vi "Get Target Train Field (No Objects).vi"(8 "Train to Field":dbl[unit]=7.0, 9 "Original Field":dbl[unit], 10 "going up?":bool=TRUE, 11 "Cluster In":T4={"Field"=0.0, "Rate"=0.0, "Status"={"Sweeping"=FALSE, "Clamped"=FALSE, "Hold"=FALSE, "At Rest"=FALSE, "Quench"=FALSE, "Persistent Mode"=FALSE, "Switch Heater"=FALSE}, "ILM Shut Down?"=FALSE, "IO Info"={"Address"={"Com Port"=1, "ISOBUS Address"=2, "GPIB Address"=24, "Communication"=enum."ISOBUS"}, "Version"=enum."IPS"}, "IO Info (Level Meter)"={"Address"={"Com Port"=1, "ISOBUS Address"=5, "GPIB Address"=24, "Communication"=enum."ISOBUS"}, "ILM Name"="", "Display Channel"=[]}, "Training?"=FALSE, "Training Field and Speed Cluster"={"Training Field"=[0.0, 4.108, 5.78, 8.001], "Training Speed"=[0.0057, 0.0022833333333333334, 0.0011333333333333334, 0.0011333333333333334]}}) -> (2 "Target Field":dbl[unit], 3 "Cluster Out":T4={"Field"=0.0, "Rate"=0.0, "Status"={"Sweeping"=FALSE, "Clamped"=FALSE, "Hold"=FALSE, "At Rest"=FALSE, "Quench"=FALSE, "Persistent Mode"=FALSE, "Switch Heater"=FALSE}, "ILM Shut Down?"=FALSE, "IO Info"={"Address"={"Com Port"=1, "ISOBUS Address"=2, "GPIB Address"=24, "Communication"=enum."ISOBUS"}, "Version"=enum."IPS"}, "IO Info (Level Meter)"={"Address"={"Com Port"=1, "ISOBUS Address"=5, "GPIB Address"=24, "Communication"=enum."ISOBUS"}, "ILM Name"="", "Display Channel"=[]}, "Training?"=FALSE, "Training Field and Speed Cluster"={"Training Field"=[0.0, 4.108, 5.78, 8.001], "Training Speed"=[0.0057, 0.0022833333333333334, 0.0011333333333333334, 0.0011333333333333334]}})   [LabVIEW 2009]
uses:
  Magnet status.ctl
  Oxford/PSSUBS.LLB/PSIO.ctl
  Oxford/BUSGEN.LLB/OxfordAddress.ctl
  Power Supply.lvclass
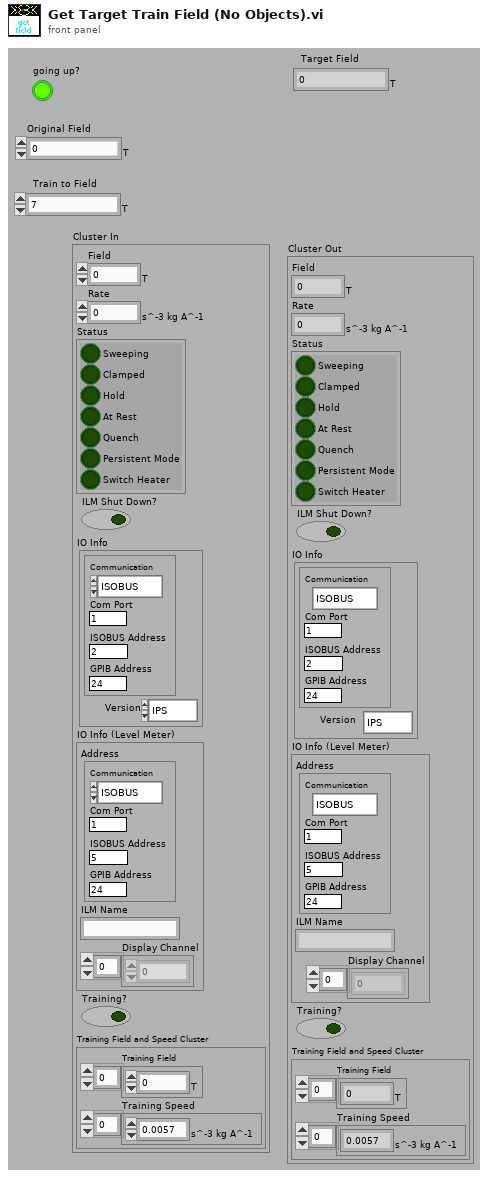
[diagram p1: front panel]
types:
  T1 = typedef "Power Supply.lvclass/Magnet status.ctl" = cluster{"Sweeping":bool, "Clamped":bool, "Hold":bool, "At Rest":bool, "Quench":bool, "Persistent Mode":bool, "Switch Heater":bool}
  T2 = typedef "PSIO.ctl" = cluster{"Address":T3, "Version":enum16{"PS", "IPS"}}
  T3 = typedef "OxfordAddress.ctl" = cluster{"Com Port":i32, "ISOBUS Address":i32, "GPIB Address":i16, "Communication":enum16{"RS232", "ISOBUS", "GPIB", "Gateway"}}
  T4 = cluster{"Field":dbl[unit], "Rate":dbl[unit], "Status":T1, "ILM Shut Down?":bool, "IO Info":T2, "IO Info (Level Meter)":cluster{"Address":T3, "ILM Name":string, "Display Channel":i32[]}, "Training?":bool, "Training Field and Speed Cluster":cluster{"Training Field":dbl[unit][], "Training Speed":dbl[unit][]}}
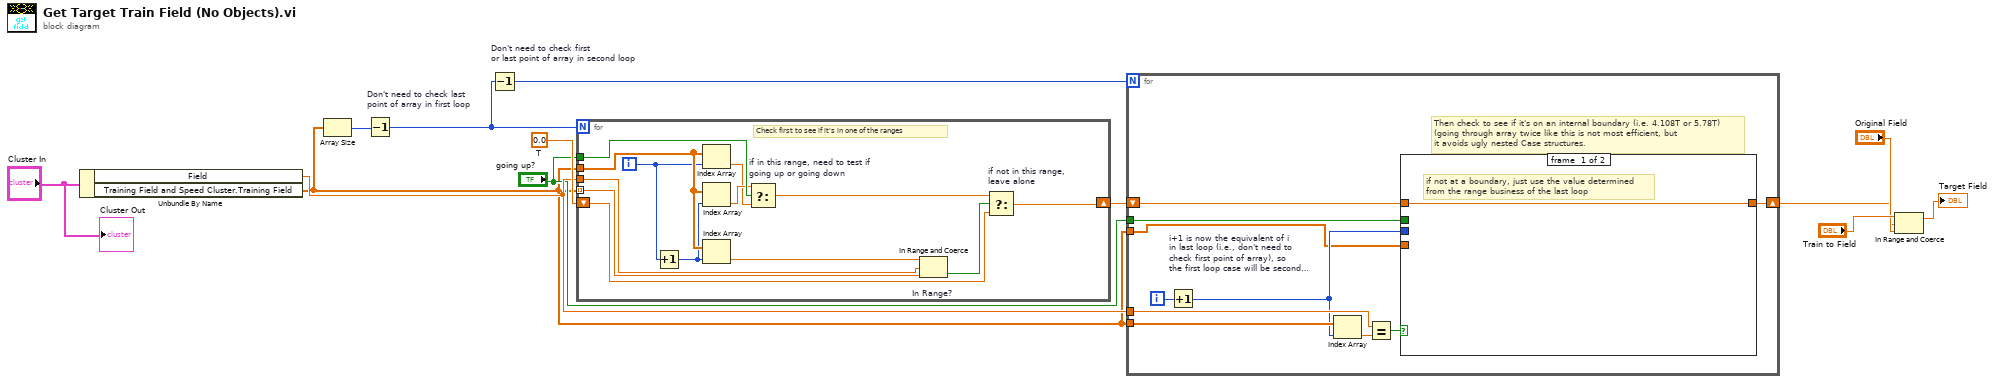
[diagram p0: block diagram]
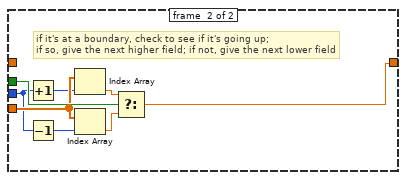
[diagram p2: hidden frame]
diagram:
  w12 = dbl[unit] 0.0  # T
  n1 = Unbundle By Name("Cluster In") -> ("Field"=w9:dbl[unit], "Training Field and Speed Cluster.Training Field"=w6:dbl[unit][])
  n2 = Array Size(array=w6) -> (size(s)=w13:i32)
  n3 = Decrement "Don't need to check last \npoint of array in first loop"(x=w13) -> (x-1=w10:i32)
  n4 = Decrement "Don't need to check first\nor last point of array in second loop"(x=w10) -> (x-1=w8:i32)
  n5 = for {
    N: w10 -> [_]
    tunnel: w9 -> [w25]
    tunnel: w6 -> [w19]
    tunnel: w6 -> [w24] mode=indexing
    shift-right: [w22] -> w11
    shift-left: w12 -> [w21]
    tunnel: "going up?" -> [w20]
    i -> [w17]
    # "Check first to see if it's in one of the ranges"
    n6 = Increment(x=w17) -> (x+1=w18:i32)
    n7 = Index Array(array=w19, index=w17) -> (element=w15:dbl[unit])
    n8 = Index Array(array=w19, index=w18) -> (element=w16:dbl[unit])
    n9 = Index Array(array=w19, index=w18) -> (element=w26:dbl[unit])
    n10 = Select "if in this range, need to test if \ngoing up or going down"(t=w16, s=w20, f=w15) -> (s? t:f=w14:dbl[unit])
    n11 = In Range and Coerce "In Range?"(upper limit=w26, x=w25, lower limit=w24) -> (In Range?=w23:bool)  [unwired: 1 out]
    n12 = Select "if not in this range,\nleave alone"(t=w14, s=w23, f=w21) -> (s? t:f=w22:dbl[unit])
  }
  n13 = for {
    N: w8 -> [_]
    tunnel: w9 -> [w33]
    tunnel: w6 -> [w31]
    shift-right: [w35] -> w2
    shift-left: w11 -> [w34]
    tunnel: "going up?" -> [w28]
    tunnel: w6 -> [w27]
    i -> [w36]
    # "Then check to see if it's on an internal boundary (i.e. 4.108T or 5.78T)\n(going through array twice like this is not most efficient, but\nit avoids ugly nested Case structures."
    n14 = Increment "i+1 is now the equivalent of i\nin last loop (i.e., don't need to \ncheck first point of array), so \nthe first loop case will be second\npoint"(x=w36) -> (x+1=w29:i32)
    n15 = Index Array(array=w31, index=w29) -> (element=w30:dbl[unit])
    n16 = Equal?(x=w33, y=w30) -> (x = y?=w32:bool)
    n17 = case shown="True" w32 {
      tunnel: [w37 w40] -> w35
      tunnel: w34 -> [w37 _]
      tunnel: w29 -> [_ w39]
      tunnel: w28 -> [_ w42]
      tunnel: w27 -> [_ w41]
      frame #0 {
        # "if not at a boundary, just use the value determined \nfrom the range business of the last loop"
      }
      frame #1 {
        # "if it's at a boundary, check to see if it's going up; \nif so, give the next higher field; if not, give the next lower field"
        n18 = Increment(x=w39) -> (x+1=w38:i32)
        n19 = Decrement(x=w39) -> (x-1=w45:i32)
        n20 = Index Array(array=w41, index=w38) -> (element=w44:dbl[unit])
        n21 = Index Array(array=w41, index=w45) -> (element=w43:dbl[unit])
        n22 = Select(t=w44, s=w42, f=w43) -> (s? t:f=w40:dbl[unit])
      }
    }
  }
  n23 = In Range and Coerce(upper limit="Train to Field", x=w2, lower limit="Original Field") -> (coerced(x)=→"Target Field":dbl[unit])  [unwired: 1 out]
  "Cluster Out" <- "Cluster In"
